vi "Numeric Toggle.vi"(10 "# of Cases":i32, 11 "Toggle Input":bool) -> (3 "Output":i32)   [LabVIEW 2016]
uses:
  <vilib>/ptbypt/NI_PtbyPt.lvlib
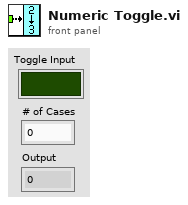
[diagram p1: front panel]
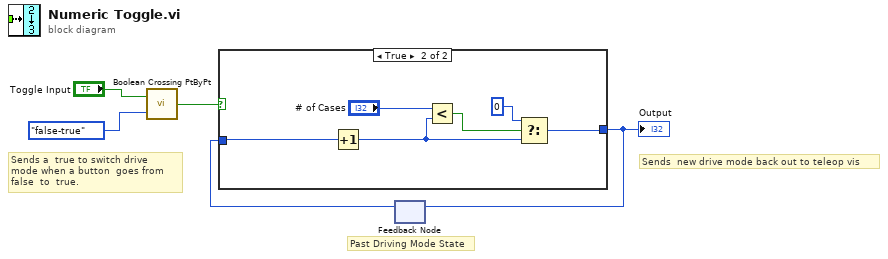
[diagram p0: block diagram]
diagram:
  # "Sends  new drive mode back out to teleop vis"
  # "Sends a  true to switch drive\nmode when a button  goes from \nfalse  to  true."
  # "Past Driving Mode State"
  n1 = call <vilib>:"Boolean Crossing PtByPt.vi"("direction"=enum16{"either", "false-true", "true-false"}."false-true", "input"="Toggle Input") -> ("crossing"=w3:bool)  [unwired: 1 in]
  n2 = feedback #1() -> (w2:i32)  [unwired: 1 in]
  n3 = case shown="True" w3 {
    tunnel: w2 -> [w6 w7]
    tunnel: [w6 w8] -> w1
    frame False {
      # "Stays the same when no change in  button state"
    }
    frame True {
      n4 = Increment(x=w7) -> (x+1=w9:i32)
      n5 = Less?(x="# of Cases", y=w9) -> (x < y?=w12:bool)
      n6 = Select(t=0, s=w12, f=w9) -> (s? t:f=w8:i32)
    }
  }
  "Output" <- w1
  n7 = feedback-in #1(w1) -> ()
